vi "Create HELLO msg (MsgPack).vi"(6 "aututhextras":string, 8 "error in (no error)":errorcluster, 9 "Authmethods":string[](array[string]), 10 "Auth ID":string, 11 "Realm":string) -> (0 "error out":errorcluster, 3 "MsgPack Bytes":u8[](array[numeric]) format="%x")   [LabVIEW 2020, in "wamplv.lvlib" / "WAMP Client.lvclass"]
uses:
  WAMP Client.lvclass
  MessagePack/MsgPackArray/MsgPackArray.lvclass
  TypeDef/WAMP Message Codes.ctl
  MessagePack/MessagePackNumeric/MessagePackNumeric.lvclass/MessagePackNumeric.ctl
  MessagePack/MsgPackMap/MsgPackMap.lvclass
  C:/local/wamplv/MessagePack/IMessagePackObject/IMessagePackObject.lvclass
  1d43950e-594c-42ae-8d22-798474962206.vi
  1d43950e-594c-42ae-8d22-798474962206.vi/43eb2b57-f62b-468b-8fb3-1a6f0340bbdf.vi
  MessagePack/MessagePackNumeric/Accessors/Write Numeric Bytes.vi
  MessagePack/MessagePackNumeric/Accessors/Write Type.vi
  MessagePack/MessagePackNumeric/MessagePackNumeric.lvclass
  MessagePack/MessagePack.lvclass
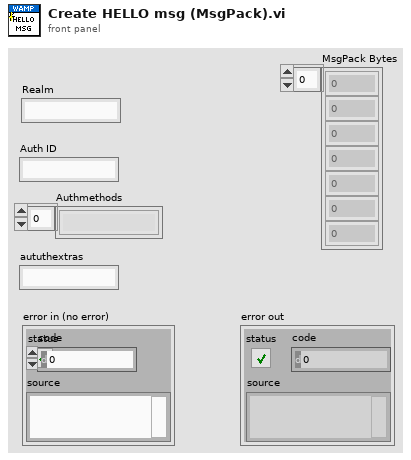
[diagram p1: front panel]
types:
  T1 = typedef "wamplv.lvlib/WAMP Client.lvclass/WAMP Message Codes.ctl" = u16
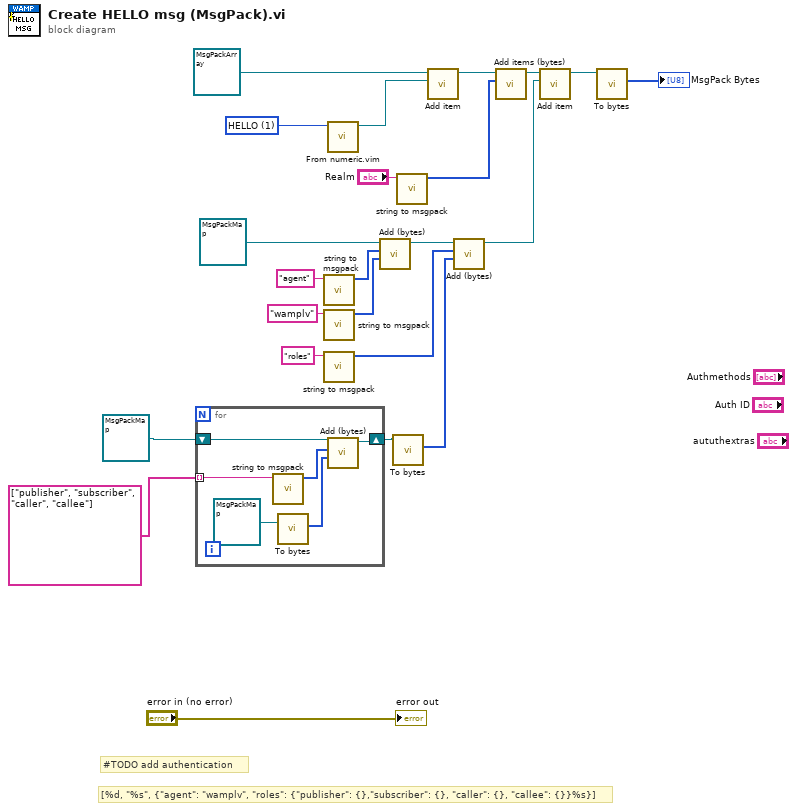
[diagram p0: block diagram]
diagram:
  w7 = T1 1 items=["HELLO"=1, "WELCOME"=2, "ABORT"=3, "GOODBYE"=6, "ERROR"=8, "PUBLISH"=16, "PUBLISHED"=17, "SUBSCRIBE"=32, "SUBSCRIBED"=33, "UNSUBSCRIBE"=34, "UNSUBSCRIBED"=35, "EVENT"=36, "CALL"=48, "RESULT"=59, "REGISTER"=64, "REGISTERED"=65, "UNREGISTER"=66, "UNREGISTERED"=67, "INVOCATION"=68, "YIELD"=70] ("Message Codes")
  # "[%d, \"%s\", {\"agent\": \"wamplv\", \"roles\": {\"publisher\": {},\"subscriber\": {}, \"caller\": {}, \"callee\": {}}%s}]"
  # "#TODO add authentication"
  n1 = for {
    tunnel: string[] ["publisher", "subscriber", "caller", "callee"] -> [w26] mode=indexing
    shift-right: [w24] -> w11
    shift-left: refnum<class "MsgPackMap.lvclass"> refnum ("wamplv.lvlib:MsgPackMap.lvclass") -> [w25]
    n2 = call "string to msgpack.vi"("String"=w26) -> ("msgpack"=w29:u8[])  [unwired: 10 in]
    n3 = call-dynamic "To bytes.vi"("MsgPackMap in"=refnum<class "MsgPackMap.lvclass"> refnum ("wamplv.lvlib:MsgPackMap.lvclass")) -> ("Array"=w27:u8[])  [unwired: 9 in, 1 out]
    n4 = call-dynamic "Add (bytes).vi"("value"=w27, "key"=w29, "MsgPackMap in"=w25) -> ("MsgPackMap out"=w24:refnum<class "MsgPackMap.lvclass">)  [unwired: 8 in]
  }
  n5 = call "string to msgpack.vi"("String"="agent") -> ("msgpack"=w18:u8[])  [unwired: 10 in]
  n6 = call "string to msgpack.vi"("String"="wamplv") -> ("msgpack"=w17:u8[])  [unwired: 10 in]
  n7 = call "string to msgpack.vi"("String"="roles") -> ("msgpack"=w14:u8[])  [unwired: 10 in]
  n8 = call "From numeric.vim"("Number"=w7) -> ("MessagePackNumeric out"=w4:refnum<class "MessagePackNumeric.lvclass">)  [unwired: 9 in, 1 out]
  n9 = call-dynamic "Add (bytes).vi"("value"=w17, "key"=w18, "MsgPackMap in"=refnum<class "MsgPackMap.lvclass"> refnum ("wamplv.lvlib:MsgPackMap.lvclass")) -> ("MsgPackMap out"=w13:refnum<class "MsgPackMap.lvclass">)  [unwired: 8 in]
  n10 = call-dynamic "To bytes.vi"("MsgPackMap in"=w11) -> ("Array"=w10:u8[])  [unwired: 9 in, 1 out]
  n11 = call "string to msgpack.vi"("String"="Realm") -> ("msgpack"=w22:u8[])  [unwired: 10 in]
  n12 = call "Add item.vi"("wamplv.lvlib:IMessagePackObject.lvclass"=w4, "MsgPackArray in"=refnum<class "MsgPackArray.lvclass"> refnum ("wamplv.lvlib:MsgPackArray.lvclass")) -> ("MsgPackArray out"=w6:refnum<class "MsgPackArray.lvclass">)  [unwired: 9 in]
  n13 = call-dynamic "Add (bytes).vi"("value"=w10, "key"=w14, "MsgPackMap in"=w13) -> ("MsgPackMap out"=w2:refnum<class "MsgPackMap.lvclass">)  [unwired: 8 in]
  n14 = call "Add items (bytes).vi"("Array"=w22, "MsgPackArray in"=w6) -> ("MsgPackArray out"=w3:refnum<class "MsgPackArray.lvclass">)  [unwired: 9 in]
  n15 = call "Add item.vi"("wamplv.lvlib:IMessagePackObject.lvclass"=w2, "MsgPackArray in"=w3) -> ("MsgPackArray out"=w1:refnum<class "MsgPackArray.lvclass">)  [unwired: 9 in]
  n16 = call-dynamic "To bytes.vi"("MsgPackArray in"=w1) -> ("Array"=→"MsgPack Bytes":u8[])  [unwired: 9 in, 1 out]
  "error out" <- "error in (no error)"
